vi "CheckNumberOfLocals.vi"(4 "error in":errorcluster, 5 "maximum number of locals":dbl, 6 "Rule Analysis Data In":refnum<k7>, 7 "AnalysisContext In":refnum<k7>) -> (0 "error out":errorcluster, 2 "Rule Analysis Data Out":refnum<k7>, 3 "AnalysisContext Out":refnum<k7>)   [LabVIEW 2011]
uses:
  CheckNumberOfLocalsRuleConstants.vi
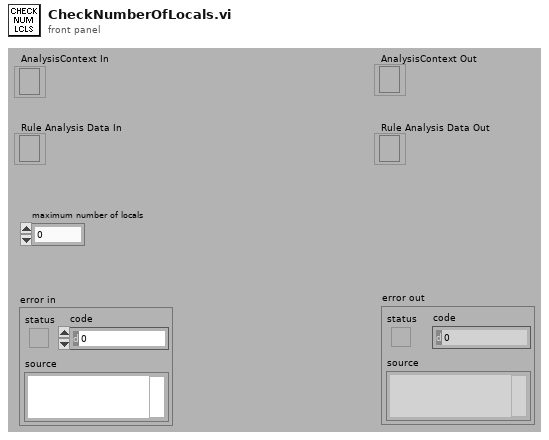
[diagram p1: front panel]
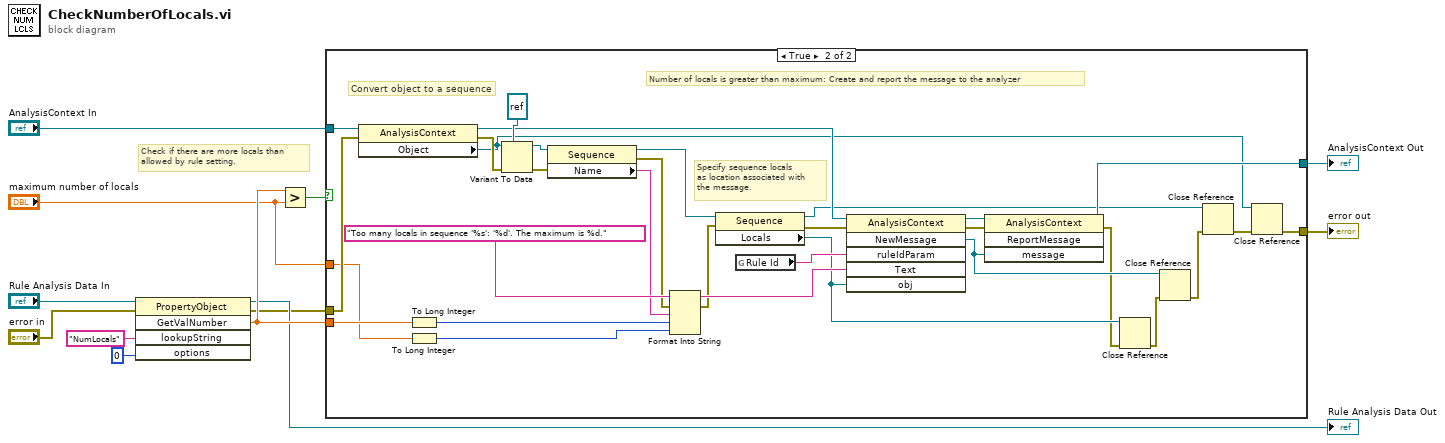
[diagram p0: block diagram]
diagram:
  # "Check if there are more locals than\nallowed by rule setting."
  n1 = invoke class="PropertyObject" method="GetValNumber"(reference="Rule Analysis Data In", error in="error in", "lookupString"="NumLocals", "options"=0) -> (reference out=→"Rule Analysis Data Out":refnum<k7>, error out=w3:errorcluster, "GetValNumber"=w12:dbl)  [unwired: 1 in, 2 out]
  n2 = Greater?(x=w12, y="maximum number of locals") -> (0:w11:bool)
  n3 = case shown="True" w11 {
    tunnel: w12 -> [_ w37]
    tunnel: [w13 w34] -> w1
    tunnel: "AnalysisContext In" -> [w14 w33]
    tunnel: [w14 w29] -> w5
    tunnel: w3 -> [w13 w28]
    tunnel: "maximum number of locals" -> [_ w27]
    frame False {
      # "Number of locals is less than maximum: Do nothing"
    }
    frame True {
      # "Specify sequence locals\nas location associated with\nthe message."
      # "Convert object to a sequence"
      # "Number of locals is greater than maximum: Create and report the message to the analyzer"
      n4 = property class="AnalysisContext"(reference=w33, error in=w28) -> (reference out=w26:refnum<k7>, error out=w32:errorcluster, "Object"=w20:refnum<k7>)
      n5 = To Long Integer(number=w37) -> (32bit integer=w36:i32)
      n6 = To Long Integer(number=w27) -> (32bit integer=w35:i32)
      n7 = Variant To Data(error in=w32, type=refnum<k7> refnum ("TS.Sequence"), Variant=w20) -> (data=w25:refnum<k7>, error out=w31:errorcluster)
      n8 = property class="Sequence"(reference=w25, error in=w31) -> (reference out=w23:refnum<k7>, error out=w38:errorcluster, "Name"=w39:string)
      n9 = Format Into String(format string="Too many locals in sequence '%s': '%d'. The maximum is %d.", error in=w38, w39, w36, w35) -> (resulting string=w44:string, error out=w24:errorcluster)  [unwired: 1 in]
      n10 = property class="Sequence"(reference=w23, error in=w24) -> (reference out=w21:refnum<k7>, error out=w22:errorcluster, "Locals"=w18:refnum<k7>)
      n11 = global read "CheckNumberOfLocalsRuleConstants.vi" "Rule Id"() -> (w41:string)
      n12 = invoke class="AnalysisContext" method="NewMessage"(reference=w26, error in=w22, "ruleIdParam"=w41, "Text"=w44, "obj"=w18) -> (reference out=w43:refnum<k7>, error out=w42:errorcluster, "NewMessage"=w19:refnum<k7>)  [unwired: 1 in, 3 out]
      n13 = invoke class="AnalysisContext" method="ReportMessage"(reference=w43, error in=w42, "message"=w19) -> (reference out=w29:refnum<k7>, error out=w17:errorcluster)  [unwired: 1 in, 2 out]
      n14 = Close Reference(reference=w18, error in (no error)=w17) -> (error out=w16:errorcluster)
      n15 = Close Reference(reference=w19, error in (no error)=w16) -> (error out=w15:errorcluster)
      n16 = Close Reference(reference=w21, error in (no error)=w15) -> (error out=w30:errorcluster)
      n17 = Close Reference(reference=w20, error in (no error)=w30) -> (error out=w34:errorcluster)
    }
  }
  "AnalysisContext Out" <- w5
  "error out" <- w1
